vi "Read Data.vi"(0 "FPEN":refnum<class "FPEN.lvclass">) -> (2 "FP Out":T3, 3 "Pane Out":T1)   [LabVIEW 2025, in "FPEN.lvclass"]
uses:
  FPEN.lvclass
  TypeDefs_Utility/Cluster_FP_Show Hide Items.ctl
  TypeDefs_Utility/ENUM_FP_Show-Hide Select.ctl
  TypeDefs_Utility/Cluster_FP_Scroll Bars Hide Show.ctl
  FPEN.lvclass/FPEN.ctl
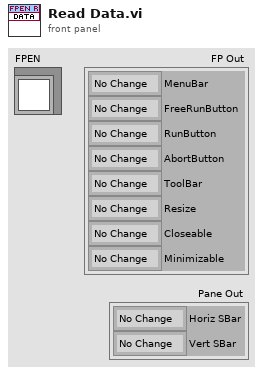
[diagram p1: front panel]
types:
  T1 = typedef "Cluster_FP_Scroll Bars Hide Show.ctl" = cluster{"Horiz SBar":T2, "Vert SBar":T2}
  T2 = typedef "ENUM_FP_Show-Hide Select.ctl" = enum16{"No Change", "Hide", "Show"}
  T3 = typedef "Cluster_FP_Show Hide Items.ctl" = cluster{"MenuBar":T2, "FreeRunButton":T2, "RunButton":T2, "AbortButton":T2, "ToolBar":T2, "Resize":T2, "Closeable":T2, "Minimizable":T2}
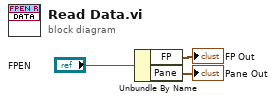
[diagram p0: block diagram]
diagram:
  n1 = Unbundle By Name("FPEN") -> ("FP"=→"FP Out":T3, "Pane"=→"Pane Out":T1)
